vi "Consumer.vi"(8 "error in (no error)":errorcluster, 9 "Data":variant, 10 "Case ID":string, 11 "uService Template in":refnum<class "TCP Listener.lvclass">) -> (0 "error out":errorcluster, 3 "uService Template out":refnum<class "TCP Listener.lvclass">)   [LabVIEW 2026, in "TALOS.lvlib" / "TCP Listener.lvlib" / "TCP Listener.lvclass"]
uses:
  TCP Listener.lvclass
  C:/LabVIEW Code/TALOS/talos/Father of all uServices/Father of all uServices/Father of all uServices.lvclass
  TCP Listener Consumer Case Selector.ctl
  Father of all uServices/Father of all uServices/Father of all uServices.lvclass/Father of all uServices.ctl
  Ancestor/Ancestor/Ancestor.lvclass/Ancestor.ctl
  TCP Listener.lvclass/TCP Listener.ctl
  Father of all uServices/Father of all uServices Messages/Consumer Msg/Consumer Msg.lvclass/Consumer Msg.ctl
  Support VIs/Generate Error.vi
  FGV/Error Memory/Get Error Description.vi
  Support VIs/Get PC name.vi
  Ancestor/Ancestor/Read ID.vi
  Support VIs/Get Class Name.vi
  FGV/Error Memory/Error Memory Core.vi
  <vilib>/AdvancedString/Delimited String to 1D String Array.vi
  <vilib>/AdvancedString/Delimited String to 1D String Array (string).vi
  Support VIs/Circus Root Path.vi
  FGV/Error Memory/Error Crt Lvl checker.vi
  FGV/Error Memory/Error Memory Core.vi/40c8088d-b597-4017-91af-faa98e00292e.vi
  FGV/Error Memory/Error Memory Core.vi/d4a3ab98-063c-4e44-b43d-fbdcfe6c2be2.vi
  Father of all uServices/Father of all uServices/Father of all uServices.lvclass
  C:/LabVIEW Code/TALOS/builds/Actor Framework PPL/Actor Framework.lvlibp/1abvi3w/vi.lib/ActorFramework/Actor/Actor.lvclass
  Support VIs/Global Memory.vi
  <vilib>/Utility/LVClass/Get LV Class Name.vi
  Support VIs/Is in Packed Library.vi
  Support VIs/TALOS Root path.vi
  Support VIs/Read CSV worksheet.vi
  Support VIs/Global Constants.vi
  <vilib>/Utility/error.llb/General Error Handler.vi
  Support VIs/Error Log.vi
  builds/Actor Framework PPL/Actor Framework.lvlibp/1abvi3w/vi.lib/ActorFramework/Actor/Read Self Enqueuer.vi
  <userlib>/_OpenG.lib/lvdata/lvdata.llb/Get Strings from Enum__ogtk.vi
  builds/Actor Framework PPL/Actor Framework.lvlibp/1abvi3w/vi.lib/ActorFramework/Message Enqueuer/Enqueue.vi
  Ancestor/Ancestor/Ancestor.lvclass
  <vilib>/Comparison/Equal/Equal Functor/Equal Functor.lvclass
  Father of all uServices/Father of all uServices Messages/Consumer Msg/Consumer Msg.lvclass
  TALOS.lvlib
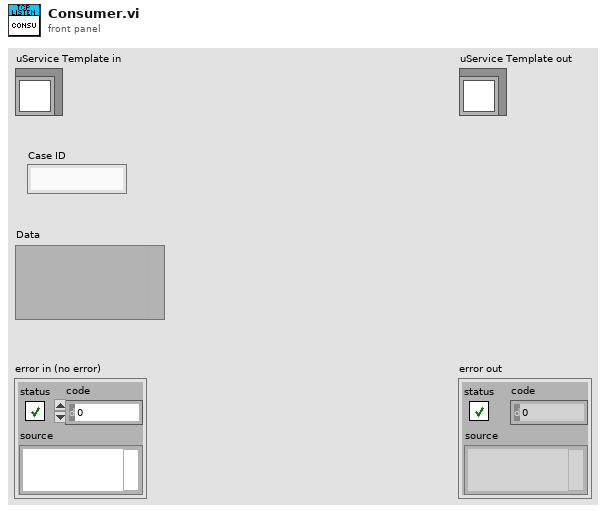
[diagram p1: front panel]
types:
  T1 = typedef "TALOS.lvlib/TCP Listener.lvlib/TCP Listener.lvclass/TCP Listener Consumer Case Selector.ctl" = enum16{"Set Client ID", "Listen", "Idle", "Start accepting connections", "Waiting for connection"}
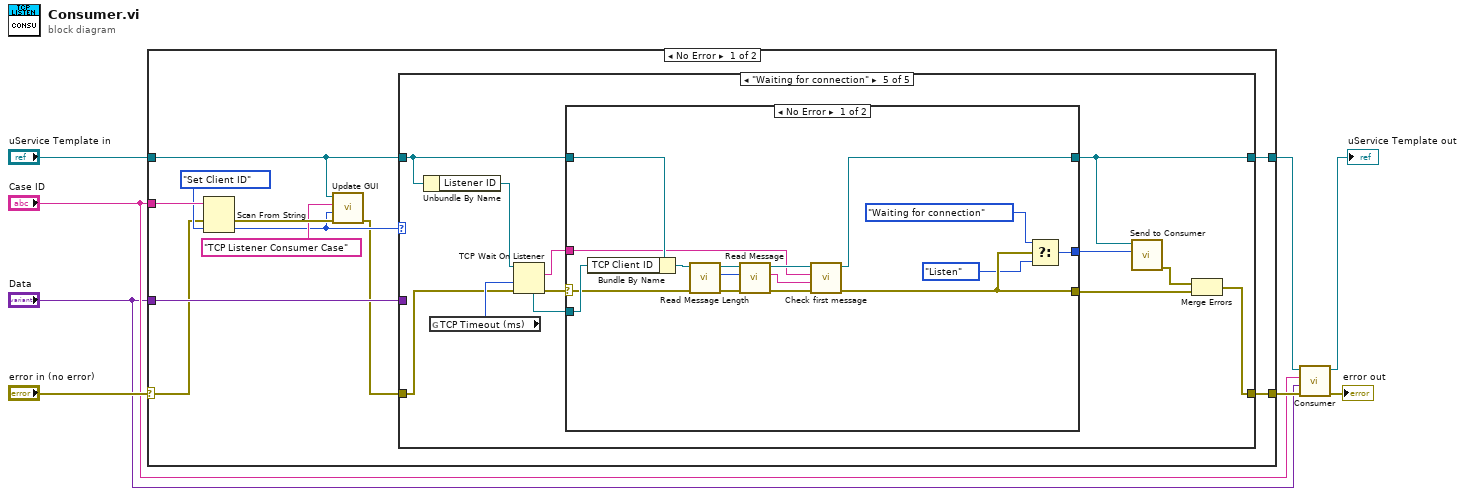
[diagram p0: block diagram]
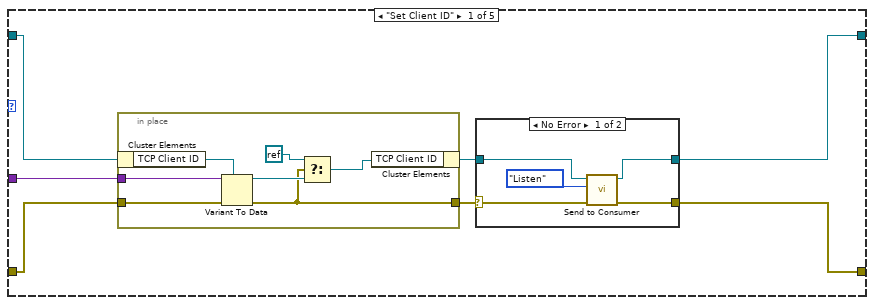
[diagram p2: hidden frame]
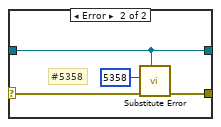
[diagram p3: hidden frame]
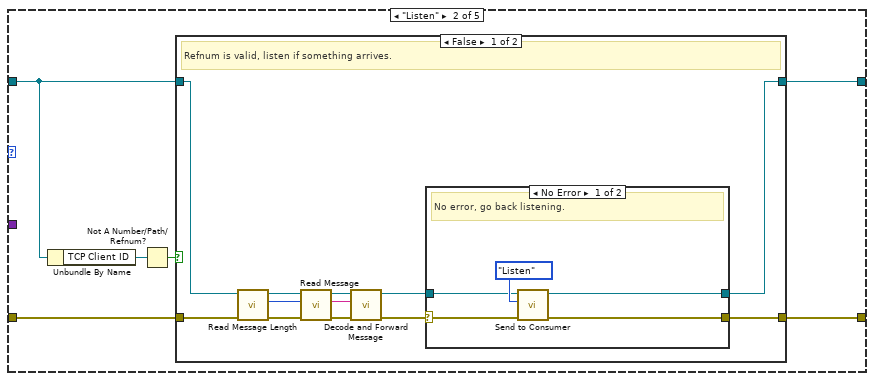
[diagram p4: hidden frame]
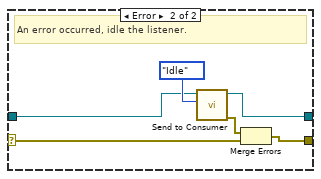
[diagram p5: hidden frame]
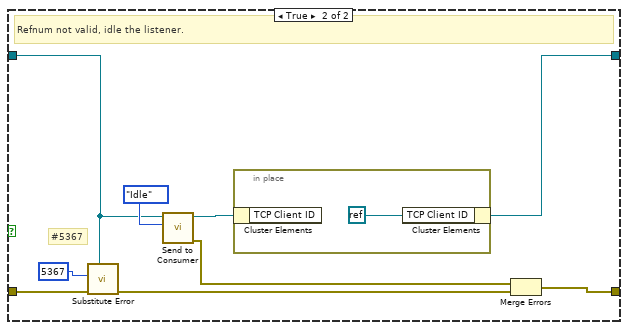
[diagram p6: hidden frame]
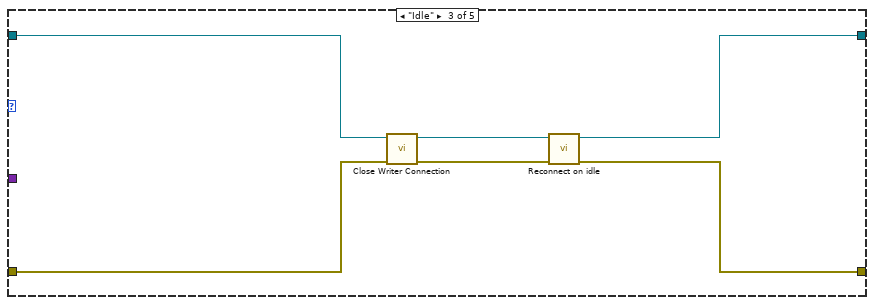
[diagram p7: hidden frame]
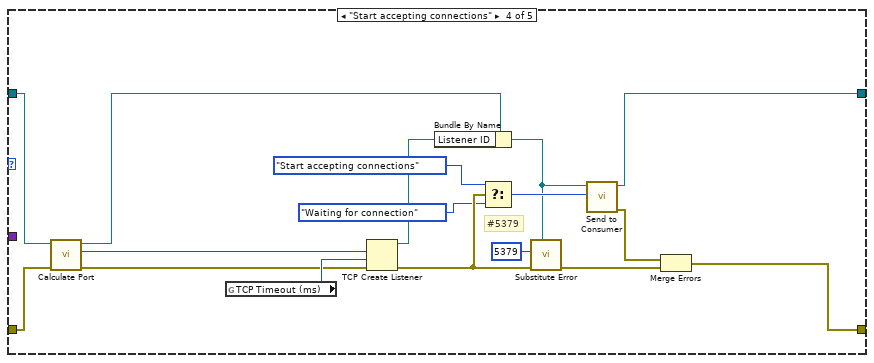
[diagram p8: hidden frame]
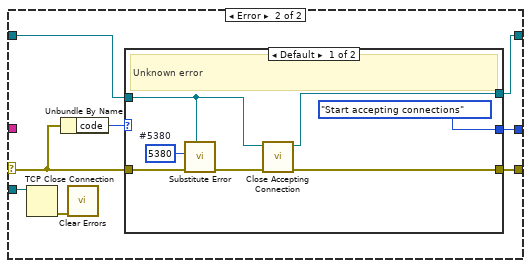
[diagram p9: hidden frame]
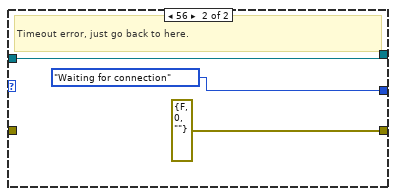
[diagram p10: hidden frame]
diagram:
  n1 = case shown="No Error" "error in (no error)" {
    selector: "error in (no error)" -> [w10 w151]
    tunnel: "uService Template in" -> [w14 w152]
    tunnel: [w17 w152] -> w4
    tunnel: [w18 w151] -> w3
    tunnel: "Case ID" -> [w16 _]
    tunnel: "Data" -> [w19 _]
    frame No Error {
      n2 = Scan From String(input string=w16, error in=w10, default 1=TCP_Listener_Consumer_Case_Selector."Set Client ID") -> (error out=w13:errorcluster, output 1=w11:T1)  [unwired: 2 in, 2 out]
      n3 = call "Update GUI.vi"("error in (no error)"=w13, "Data"=w11, "GUI Item Name"="TCP Listener Consumer Case", "uService Template in"=w14) -> ("error out"=w9:errorcluster)  [unwired: 6 in, 1 out]
      n4 = case shown="\"Waiting for connection\"" w11 {
        tunnel: w19 -> [w26 _ _ _ _]
        tunnel: w14 -> [w25 w47 w87 w104 w111]
        tunnel: [w23 w48 w82 w88 w107] -> w18
        tunnel: [w21 w46 w84 w91 w110] -> w17
        tunnel: w9 -> [w20 w43 w86 w103 w114]
        frame "Set Client ID" {
          n5 = in-place "In Place Element Structure" {
            in-place-border: w26 -> [w42]
            in-place-border: w20 -> [w41]
            in-place-border: [w37] -> w24
            n6 = in-place-cluster #1(w25) -> ("TCP Client ID"=w38:refnum<k5>)
            n7 = Variant To Data(error in=w41, type=w38, Variant=w42) -> (data=w40:refnum<k5>, error out=w37:errorcluster)
            n8 = Select(t=refnum<k0> refnum, s=w37, f=w40) -> (s? t:f=w39:refnum<k5>)
            n9 = in-place-cluster #1("TCP Client ID"=w39) -> (w22:refnum<class "TCP Listener.lvclass">)
          }
          n10 = case shown="No Error" w24 {
            selector: w24 -> [w30 w34]
            tunnel: [w29 w33] -> w23
            tunnel: w22 -> [w28 w32]
            tunnel: [w27 w32] -> w21
            frame No Error {
              n11 = call "Send to Consumer.vi"("error in (no error)"=w30, "Case ID"=TCP_Listener_Consumer_Case_Selector."Listen" ("TCP Listener Consumer Case Selector"), "uService Template in"=w28) -> ("error out"=w29:errorcluster, "uService Template out"=w27:refnum<class "TCP Listener.lvclass">)  [unwired: 7 in]
            }
            frame Error {
              # "#5358"
              n12 = call "Substitute Error.vi"("LabVIEW Object"=w32, "error in (no error)"=w34, "Error Code"=5358) -> ("error out"=w33:errorcluster)  [unwired: 8 in]
            }
          }
        }
        frame "Listen" {
          n13 = Unbundle By Name(w47) -> ("TCP Client ID"=w45:refnum<k5>)
          n14 = Not A Number/Path/Refnum?(number/path/refnum=w45) -> (NaN/Path/Refnum?=w44:bool)
          n15 = case shown="False" w44 {
            tunnel: w43 -> [w60 w76]
            tunnel: [w53 w78] -> w48
            tunnel: w47 -> [w59 w75]
            tunnel: [w50 w72] -> w46
            frame False {
              # "Refnum is valid, listen if something arrives."
              n16 = call-dynamic "Read Message Length.vi"("error in (no error)"=w60, "TCP Listener in"=w59) -> ("error out"=w57:errorcluster, "Bytes to read"=w56:i32, "TCP Listener out"=w58:refnum<class "TCP Listener.lvclass">)  [unwired: 7 in]
              n17 = call-dynamic "Read Message.vi"("error in (no error)"=w57, "Bytes to read"=w56, "TCP Listener in"=w58) -> ("error out"=w51:errorcluster, "Message string"=w49:string, "TCP Listener out"=w52:refnum<class "TCP Listener.lvclass">)  [unwired: 6 in]
              n18 = call-dynamic "Decode and Forward Message.vi"("error in (no error)"=w51, "Message undecoded"=w49, "TCP Listener in"=w52) -> ("error out"=w55:errorcluster, "TCP Listener out"=w54:refnum<class "TCP Listener.lvclass">)  [unwired: 7 in]
              n19 = case shown="No Error" w55 {
                selector: w55 -> [w64 w68]
                tunnel: w54 -> [w63 w70]
                tunnel: [w62 w67] -> w53
                tunnel: [w61 w66] -> w50
                frame No Error {
                  # "No error, go back listening."
                  n20 = call "Send to Consumer.vi"("error in (no error)"=w64, "Case ID"=TCP_Listener_Consumer_Case_Selector."Listen" ("TCP Listener Consumer Case Selector"), "uService Template in"=w63) -> ("error out"=w62:errorcluster, "uService Template out"=w61:refnum<class "TCP Listener.lvclass">)  [unwired: 7 in]
                }
                frame Error {
                  # "An error occurred, idle the listener."
                  n21 = call "Send to Consumer.vi"("Case ID"=TCP_Listener_Consumer_Case_Selector."Idle" ("TCP Listener Consumer Case Selector"), "uService Template in"=w70) -> ("error out"=w69:errorcluster, "uService Template out"=w66:refnum<class "TCP Listener.lvclass">)  [unwired: 8 in]
                  n22 = Merge Errors(w69, w68) -> (w67:errorcluster)
                }
              }
            }
            frame True {
              # "#5367"
              # "Refnum not valid, idle the listener."
              n23 = call "Substitute Error.vi"("LabVIEW Object"=w75, "error in (no error)"=w76, "Error Code"=5367) -> ("error out"=w77:errorcluster)  [unwired: 8 in]
              n24 = call "Send to Consumer.vi"("Case ID"=TCP_Listener_Consumer_Case_Selector."Idle" ("TCP Listener Consumer Case Selector"), "uService Template in"=w75) -> ("error out"=w79:errorcluster, "uService Template out"=w73:refnum<class "TCP Listener.lvclass">)  [unwired: 8 in]
              n25 = in-place {
                n26 = in-place-cluster #2(w73) -> ()  [unwired: 1 out]
                n27 = in-place-cluster #2("TCP Client ID"=refnum<k0> refnum) -> (w72:refnum<class "TCP Listener.lvclass">)
              }
              n28 = Merge Errors(w79, w77) -> (w78:errorcluster)
            }
          }
        }
        frame "Idle" {
          n29 = call-dynamic "Close Writer Connection.vi"("error in"=w86, "uService Template in"=w87) -> ("error out"=w83:errorcluster, "uService Template out"=w85:refnum<class "TCP Listener.lvclass">)  [unwired: 8 in]
          n30 = call-dynamic "Reconnect on idle.vi"("error in (no error)"=w83, "TCP Listener in"=w85) -> ("error out"=w82:errorcluster, "TCP Listener out"=w84:refnum<class "TCP Listener.lvclass">)  [unwired: 8 in]
        }
        frame "Start accepting connections" {
          # "#5379"
          n31 = call-dynamic "Calculate Port.vi"("error in (no error)"=w103, "TCP Listener in"=w104) -> ("error out"=w97:errorcluster, "Port"=w96:u16, "TCP Listener out"=w93:refnum<class "TCP Listener.lvclass">)  [unwired: 7 in]
          n32 = global read "Global Constants.vi" "TCP Timeout (ms)"() -> (w98:i32)
          n33 = TCP Create Listener(8:w97, 9:w98, 10:w96) -> (0:w102:errorcluster, 3:w100:refnum<k5>)  [unwired: 2 in, 1 out]
          n34 = Bundle By Name(cluster=w93, "Listener ID"=w100) -> (w92:refnum<class "TCP Listener.lvclass">)
          n35 = Select(t=TCP_Listener_Consumer_Case_Selector."Start accepting connections", s=w102, f=TCP_Listener_Consumer_Case_Selector."Waiting for connection") -> (s? t:f=w101:T1)
          n36 = call "Substitute Error.vi"("LabVIEW Object"=w92, "error in (no error)"=w102, "Error Code"=5379) -> ("error out"=w90:errorcluster)  [unwired: 8 in]
          n37 = call "Send to Consumer.vi"("Case ID"=w101, "uService Template in"=w92) -> ("error out"=w89:errorcluster, "uService Template out"=w91:refnum<class "TCP Listener.lvclass">)  [unwired: 8 in]
          n38 = Merge Errors(w89, w90) -> (w88:errorcluster)
        }
        frame "Waiting for connection" {
          n39 = Unbundle By Name(w111) -> ("Listener ID"=w116:refnum<k5>)
          n40 = global read "Global Constants.vi" "TCP Timeout (ms)"() -> (w115:i32)
          n41 = TCP Wait On Listener(8:w114, 9:w115, 11:w116) -> (0:w113:errorcluster, 2:w106:string, 4:w112:refnum<k5>)  [unwired: 1 in, 2 out]
          n42 = case shown="No Error" w113 {
            selector: w113 -> [w126 w138]
            tunnel: w112 -> [w128 w137]
            tunnel: w111 -> [w129 w136]
            tunnel: [w117 w133] -> w110
            tunnel: [w121 w135] -> w108
            tunnel: w106 -> [w124 _]
            tunnel: [w118 w134] -> w105
            frame No Error {
              n43 = Bundle By Name(cluster=w129, "TCP Client ID"=w128) -> (w127:refnum<class "TCP Listener.lvclass">)
              n44 = call-dynamic "Read Message Length.vi"("error in (no error)"=w126, "TCP Listener in"=w127) -> ("error out"=w131:errorcluster, "Bytes to read"=w130:i32, "TCP Listener out"=w132:refnum<class "TCP Listener.lvclass">)  [unwired: 7 in]
              n45 = call-dynamic "Read Message.vi"("error in (no error)"=w131, "Bytes to read"=w130, "TCP Listener in"=w132) -> ("error out"=w122:errorcluster, "Message string"=w123:string, "TCP Listener out"=w125:refnum<class "TCP Listener.lvclass">)  [unwired: 6 in]
              n46 = call-dynamic "Check first message.vi"("error in (no error)"=w122, "First Message"=w123, "Remote Address"=w124, "TCP Listener in"=w125) -> ("error out"=w121:errorcluster, "TCP Listener out"=w117:refnum<class "TCP Listener.lvclass">)  [unwired: 6 in]
              n47 = Select(t=TCP_Listener_Consumer_Case_Selector."Waiting for connection", s=w121, f=TCP_Listener_Consumer_Case_Selector."Listen") -> (s? t:f=w118:T1)
            }
            frame Error {
              n48 = TCP Close Connection(connection ID=w137) -> (error out=w139:errorcluster)  [unwired: 2 in, 1 out]
              n49 = Unbundle By Name(w138) -> ("code"=w140:i32)
              n50 = call <vilib>:"Clear Errors.vi"("error in (no error)"=w139) -> ()  [unwired: 5 in, 2 out]
              n51 = case shown="Default" w140 {
                tunnel: [w141 errorcluster {"status"=FALSE, "code"=0, "source"=""} ("error IO")] -> w135
                tunnel: w138 -> [w147 _]
                tunnel: w136 -> [w143 w148]
                tunnel: [TCP_Listener_Consumer_Case_Selector."Start accepting connections" TCP_Listener_Consumer_Case_Selector."Waiting for connection"] -> w134
                tunnel: [w142 w148] -> w133
                frame Default {
                  w146 = 5380  # #5380
                  # "Unknown error"
                  n52 = call "Substitute Error.vi"("LabVIEW Object"=w143, "error in (no error)"=w147, "Error Code"=w146) -> ("error out"=w144:errorcluster)  [unwired: 8 in]
                  n53 = call-dynamic "Close Accepting Connection.vi"("error in"=w144, "uService Template in"=w143) -> ("error out"=w141:errorcluster, "uService Template out"=w142:refnum<class "TCP Listener.lvclass">)  [unwired: 8 in]
                }
                frame 56 {
                  # "Timeout error, just go back to here."
                }
              }
            }
          }
          n54 = call "Send to Consumer.vi"("Case ID"=w105, "uService Template in"=w110) -> ("error out"=w109:errorcluster)  [unwired: 8 in, 1 out]
          n55 = Merge Errors(w109, w108) -> (w107:errorcluster)
        }
      }
    }
    frame Error {
    }
  }
  n56 = call-parent "Consumer.vi"("error in (no error)"=w3, "Data"="Data", "Case ID"="Case ID", "uService Template in"=w4) -> ("error out"=→"error out":errorcluster, "uService Template out"=→"uService Template out":refnum<class "TCP Listener.lvclass">)  [unwired: 6 in]
